vi "Send Message.vi"(8 "error in (no error)":errorcluster, 11 "Notify with Message in":refnum<class "Notify with Message.lvclass">) -> (0 "error out":errorcluster, 3 "Notify with Message out":refnum<class "Notify with Message.lvclass">)   [LabVIEW 2023, in "Notify with Message.lvclass"]
uses:
  Notify with Message.lvclass
  Message Data/Number/Number.lvclass
  C:/Users/Ancy.Augustin/Desktop/Sender Receiver/Classes/Message Data/Message Data.lvclass
  Controls/User Event Operations.ctl
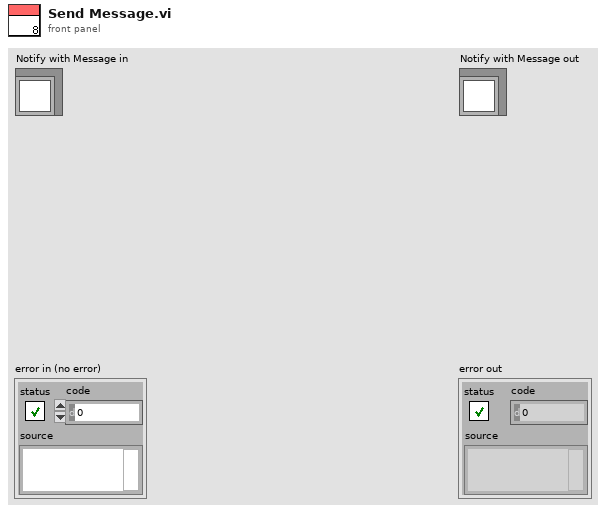
[diagram p1: front panel]
types:
  T1 = typedef "User Event Operations.ctl" = enum16{"Obtain", "Generate", "Destroy"}
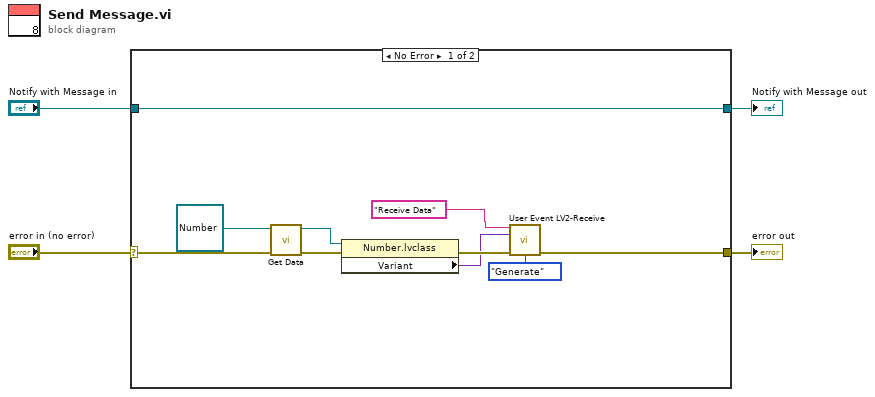
[diagram p0: block diagram]
diagram:
  n1 = case shown="No Error" "error in (no error)" {
    selector: "error in (no error)" -> [w14 w16]
    tunnel: [w8 w16] -> w3
    tunnel: [w13 w15] -> w1
    tunnel: "Notify with Message in" -> [w13 w15]
    frame No Error {
      n2 = call-dynamic "Get Data.vi"("error in (no error)"=w14, "Number in"=refnum<class "Number.lvclass"> refnum ("Number.lvclass")) -> ("error out"=w12:errorcluster, "Number out"=w9:refnum<class "Number.lvclass">)  [unwired: 8 in]
      n3 = property class="Number.lvclass"(reference=w9, error in=w12) -> (error out=w10:errorcluster, "Variant"=w7:variant)  [unwired: 1 out]
      n4 = call "User Event LV2-Receive.vi"("Event Name"="Receive Data", "Data"=w7, "Error In"=w10, "Operation"=User_Event_Operations."Generate") -> ("Error Out"=w8:errorcluster)  [unwired: 10 in, 1 out]
    }
    frame Error {
    }
  }
  "error out" <- w3
  "Notify with Message out" <- w1
